vi "Update UI.vi"(0 "Serial port assistant view in":refnum<class "Serial port assistant view.lvclass">, 7 "changed data":string, 11 "error in (no error)":errorcluster) -> (4 "Serial port assistant view out":refnum<class "Serial port assistant view.lvclass">, 15 "error out":errorcluster)   [LabVIEW 2022 SP3, in "Serial port assistant view.lvlib" / "Serial port assistant view.lvclass"]
uses:
  Serial port assistant view.lvclass
  serial port list--type.ctl
  Serial port assistant view.lvclass/Serial port assistant view.ctl
  data has been sent--type.ctl
  data has been received--type.ctl
  serial port status--type.ctl
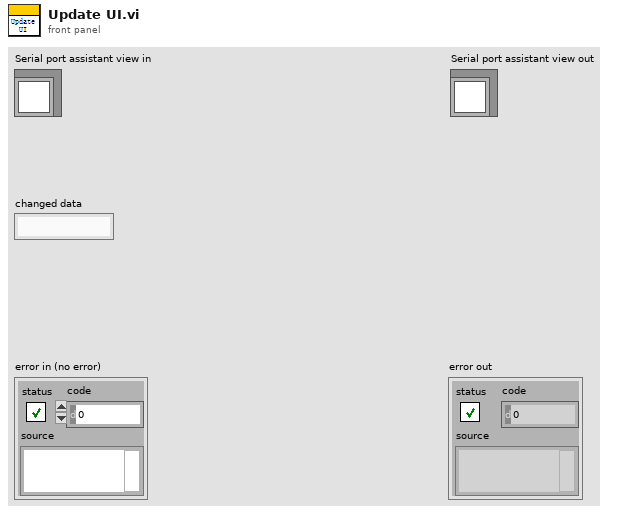
[diagram p1: front panel]
types:
  T1 = typedef "Serial port assistant view.lvlib/Serial port assistant view.lvclass/serial port list--type.ctl" = cluster{"serial port list":string[]}
  T2 = typedef "Serial port assistant view.lvlib/Serial port assistant view.lvclass/serial port status--type.ctl" = cluster{"serial port":string, "baud rate":u32, "data bits":u16, "stop bits":u16, "parity":u16, "open":bool}
  T3 = typedef "Serial port assistant view.lvlib/Serial port assistant view.lvclass/data has been sent--type.ctl" = cluster{"send time":string, "data has been sent":string}
  T4 = typedef "Serial port assistant view.lvlib/Serial port assistant view.lvclass/data has been received--type.ctl" = cluster{"receive time":string, "data has been received":string}
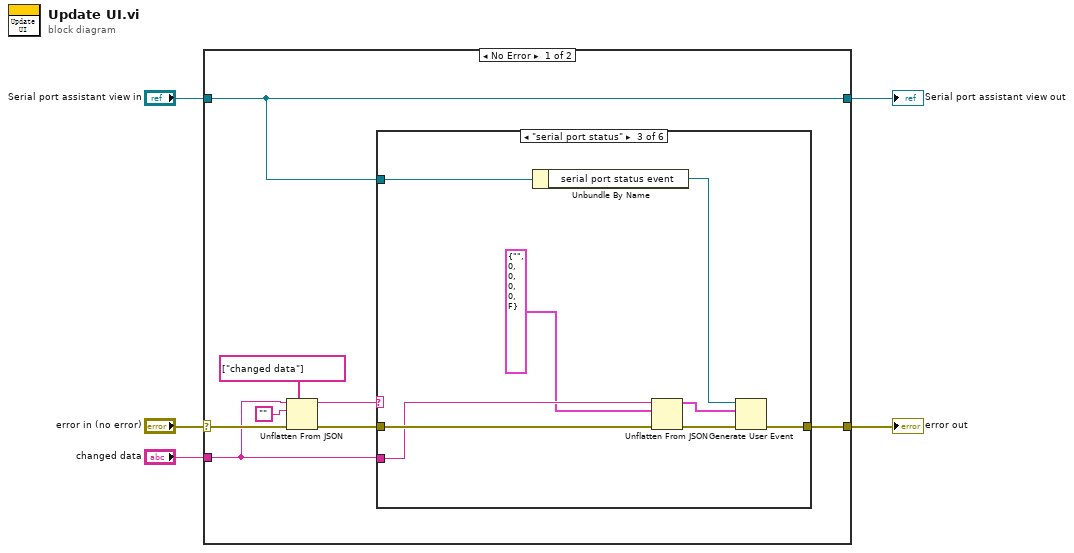
[diagram p0: block diagram]
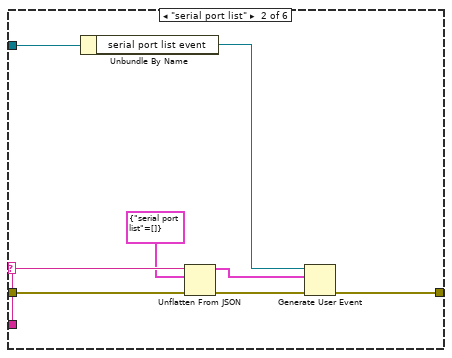
[diagram p3: hidden frame]
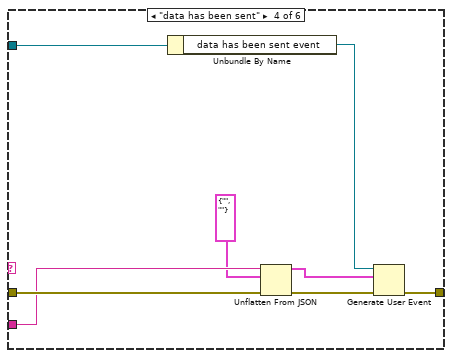
[diagram p4: hidden frame]
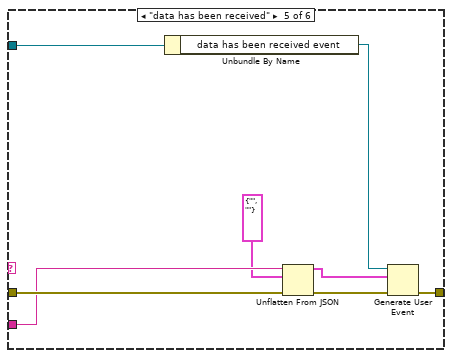
[diagram p5: hidden frame]
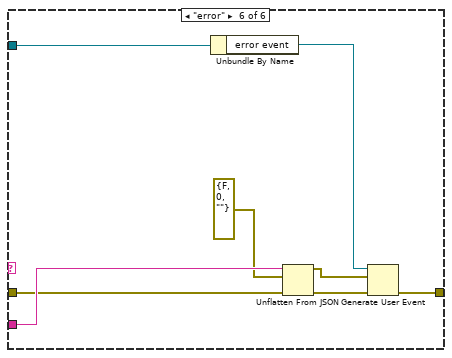
[diagram p6: hidden frame]
diagram:
  n1 = case shown="No Error" "error in (no error)" {
    selector: "error in (no error)" -> [w12 w55]
    tunnel: [w9 w55] -> w4
    tunnel: "Serial port assistant view in" -> [w7 w56]
    tunnel: [w7 w56] -> w2
    tunnel: "changed data" -> [w8 _]
    frame No Error {
      n2 = Unflatten From JSON(path=string[] ["changed data"], JSON string=w8, type and defaults="", error in (no error)=w12) -> (value=w11:string, error out=w10:errorcluster)  [unwired: 3 in]
      n3 = case shown="\"serial port status\"" w11 {
        tunnel: w10 -> [w14 w22 w30 w38 w46 w49]
        tunnel: [w14 w15 w24 w33 w41 w50] -> w9
        tunnel: w8 -> [_ w21 w29 w37 w45 w54]
        tunnel: w7 -> [_ w18 w27 w35 w43 w52]
        frame "null", Default {
        }
        frame "serial port list" {
          n4 = Unbundle By Name(w18) -> ("serial port list event"=w17:refnum<user-event>)
          n5 = Unflatten From JSON(JSON string=w21, type and defaults=T1 {"serial port list"=[]} ("serial port list"), error in (no error)=w22) -> (value=w16:T1, error out=w19:errorcluster)  [unwired: 4 in]
          n6 = Generate User Event(user event=w17, event data cluster=w16, error in=w19) -> (error out=w15:errorcluster)  [unwired: 1 in, 1 out]
        }
        frame "serial port status" {
          n7 = Unbundle By Name(w27) -> ("serial port status event"=w26:refnum<user-event>)
          n8 = Unflatten From JSON(JSON string=w29, type and defaults=T2 {"serial port"="", "baud rate"=0, "data bits"=0, "stop bits"=0, "parity"=0, "open"=FALSE} ("serial port status"), error in (no error)=w30) -> (value=w25:T2, error out=w28:errorcluster)  [unwired: 4 in]
          n9 = Generate User Event(user event=w26, event data cluster=w25, error in=w28) -> (error out=w24:errorcluster)  [unwired: 1 in, 1 out]
        }
        frame "data has been sent" {
          n10 = Unbundle By Name(w35) -> ("data has been sent event"=w34:refnum<user-event>)
          n11 = Unflatten From JSON(JSON string=w37, type and defaults=T3 {"send time"="", "data has been sent"=""} ("data has been sent"), error in (no error)=w38) -> (value=w31:T3, error out=w36:errorcluster)  [unwired: 4 in]
          n12 = Generate User Event(user event=w34, event data cluster=w31, error in=w36) -> (error out=w33:errorcluster)  [unwired: 1 in, 1 out]
        }
        frame "data has been received" {
          n13 = Unbundle By Name(w43) -> ("data has been received event"=w42:refnum<user-event>)
          n14 = Unflatten From JSON(JSON string=w45, type and defaults=T4 {"receive time"="", "data has been received"=""} ("data has been received"), error in (no error)=w46) -> (value=w39:T4, error out=w44:errorcluster)  [unwired: 4 in]
          n15 = Generate User Event(user event=w42, event data cluster=w39, error in=w44) -> (error out=w41:errorcluster)  [unwired: 1 in, 1 out]
        }
        frame "error" {
          n16 = Unbundle By Name(w52) -> ("error event"=w51:refnum<user-event>)
          n17 = Unflatten From JSON(JSON string=w54, type and defaults=errorcluster {"status"=FALSE, "code"=0, "source"=""} ("error out"), error in (no error)=w49) -> (value=w48:errorcluster, error out=w53:errorcluster)  [unwired: 4 in]
          n18 = Generate User Event(user event=w51, event data cluster=w48, error in=w53) -> (error out=w50:errorcluster)  [unwired: 1 in, 1 out]
        }
      }
    }
    frame Error {
    }
  }
  "error out" <- w4
  "Serial port assistant view out" <- w2
